vi "StringToBooleanArray(cast).vi"(1 "Str":string) -> (0 "U8[]":u8[](array[numeric]))   [LabVIEW 2012]
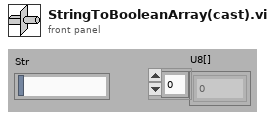
[diagram p1: front panel]
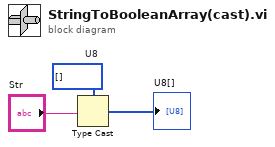
[diagram p0: block diagram]
diagram:
  w2 = u8[] []  # U8
  n1 = Type Cast(type=w2, x="Str") -> (*(type *) &x=→"U8[]":u8[])
